vi "Open Shared Memory File.vi"(7 "permissions (0664)":T1={"owner"={"read"=TRUE, "write"=TRUE, "execute"=FALSE}, "group"={"read"=TRUE, "write"=TRUE, "execute"=FALSE}, "everyone"={"read"=TRUE, "write"=FALSE, "execute"=FALSE}}, 8 "error in (no error)":errorcluster, 9 "file mode (open)":T3, 10 "access mode (read and write)":enum16{"read only", "read and write"}(ring)=enum."read and write", 11 "shared memory name":string="temp") -> (0 "error out":errorcluster, 3 "shared memory out":T2)   [LabVIEW 2013, in "Linux RT IPC.lvlib" / "Shared Memory.lvlib" / "Shared Memory.lvclass"]
doc: "This VI creates a new shared memory file or opens a reference to an exisitng shared memory file created by another process. The shared memory name follows the format of \"/<name>\", rather than using a full path such as /dev/shm/<name>. This allows for the location of shared memory to be relocated by the operating system without requiring the application to know the exact path. The user can also set the access permissions of the shared memory according to the needs of the application."
uses:
  Shared Memory.lvclass
  Controls/file mode.ctl
  Controls/reference.ctl
  Shared Memory.lvclass/Shared Memory.ctl
  Shared Memory.lvlib
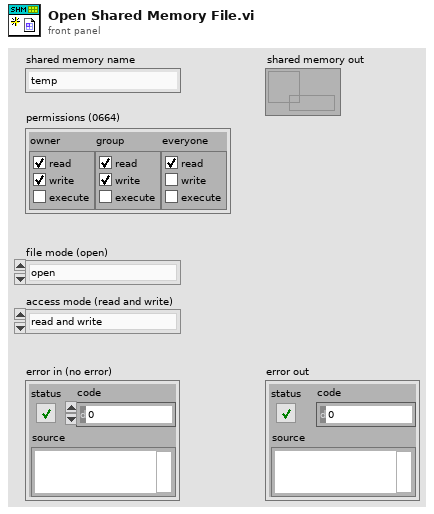
[diagram p1: front panel]
types:
  T1 = cluster{"owner":cluster{"read":bool, "write":bool, "execute":bool}, "group":cluster{"read":bool, "write":bool, "execute":bool}, "everyone":cluster{"read":bool, "write":bool, "execute":bool}}
  T2 = typedef "Linux RT IPC.lvlib/Shared Memory.lvlib/reference.ctl" = refnum<data-value>
  T3 = typedef "Linux RT IPC.lvlib/Shared Memory.lvlib/file mode.ctl" = enum16{"open", "create/replace"}
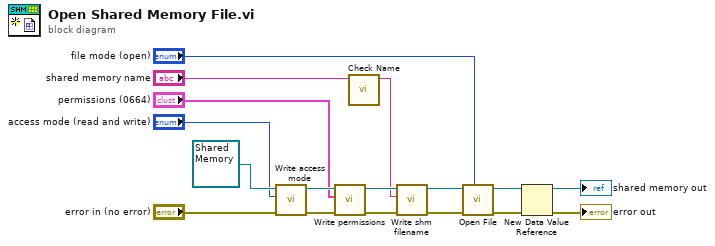
[diagram p0: block diagram]
diagram:
  n1 = call "Write access mode.vi"("error in (no error)"="error in (no error)", "access mode"="access mode (read and write)", "Shared Memory in"=refnum<class "Shared Memory.lvclass"> refnum ("Shared Memory.lvlib:Shared Memory")) -> ("error out"=w11:errorcluster, "Shared Memory out"=w10:refnum<class "Shared Memory.lvclass">)  [unwired: 7 in]
  n2 = call "Write permissions.vi"("error in (no error)"=w11, "permissions"="permissions (0664)", "Shared Memory in"=w10) -> ("error out"=w8:errorcluster, "Shared Memory out"=w9:refnum<class "Shared Memory.lvclass">)  [unwired: 7 in]
  n3 = call "Check Name.vi"("shared memory name in"="shared memory name") -> ("shared memory name out"=w6:string)  [unwired: 10 in]
  n4 = call "Write shm filename.vi"("error in (no error)"=w8, "shm filename"=w6, "Shared Memory in"=w9) -> ("error out"=w4:errorcluster, "Shared Memory out"=w5:refnum<class "Shared Memory.lvclass">)  [unwired: 7 in]
  n5 = call "Open File.vi"("file mode"="file mode (open)", "error in (no error)"=w4, "Shared Memory in"=w5) -> ("error out"=w1:errorcluster, "Shared Memory out"=w2:refnum<class "Shared Memory.lvclass">)  [unwired: 7 in]
  n6 = New Data Value Reference(data value=w2, error in=w1) -> (data value reference=→"shared memory out":refnum<data-value>, error out=→"error out":errorcluster)
